vi "Measure_Voltage.vi"(6 "Resolution in Digits":T1(ring), 8 "error in (no error)":errorcluster, 9 "Range":dbl=1.2, 10 "Level":dbl=1.2, 11 "NI-DMM in":refnum<class "niDMM.lvclass">) -> (0 "error out":errorcluster, 1 "Out of Range":bool, 2 "DC_Voltage":dbl, 3 "NI-DMM out":refnum<class "niDMM.lvclass">)   [LabVIEW 2021, in "niDMM.lvclass"]
uses:
  niDMM.lvclass
  niDMM.lvclass/niDMM.ctl
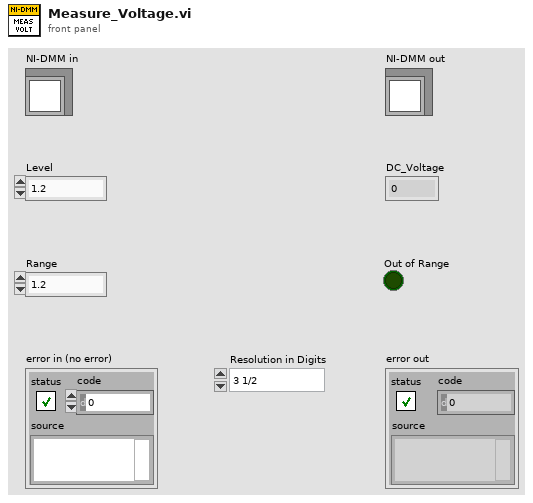
[diagram p1: front panel]
types:
  T1 = enum32{"3 1/2", "4 1/2", "5 1/2", "6 1/2", "7 1/2"}
  T2 = enum32{"DC Volts", "AC Volts", "DC Current", "AC Current", "2-wire Resistance", "4-wire Resistance", "Diode", "Frequency", "Period", "AC Volts DC Coupled", "Capacitance", "Inductance", "Temperature"}
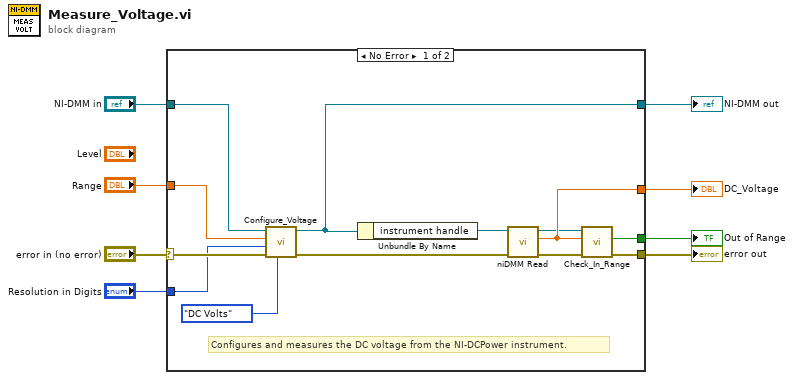
[diagram p0: block diagram]
diagram:
  n1 = case shown="No Error" "error in (no error)" {
    selector: "error in (no error)" -> [w21 w22]
    tunnel: "NI-DMM in" -> [w20 w23]
    tunnel: [w19 w22] -> w6
    tunnel: [w18 _] -> w5
    tunnel: [w15 w23] -> w4
    tunnel: [w16 _] -> w3
    tunnel: "Range" -> [w11 _]
    tunnel: "Resolution in Digits" -> [w10 _]
    frame No Error {
      # "Configures and measures the DC voltage from the NI-DCPower instrument."
      n2 = call-dynamic "Configure_Voltage.vi"("Measurement Type"=T2."DC Volts", "error in (no error)"=w21, "Resolution in Digits"=w10, "Range"=w11, "NI-DMM in"=w20) -> ("error out"=w17:errorcluster, "NI-DMM out"=w15:refnum<class "niDMM.lvclass">)  [unwired: 5 in]
      n3 = Unbundle By Name(w15) -> ("instrument handle"=w14:refnum<k15>)
      n4 = call <instrlib>:"niDMM Read.vi"("error in (no error)"=w17, "instrument handle"=w14) -> ("error out"=w12:errorcluster, "Measurement"=w18:dbl, "instrument handle out"=w13:refnum<k15>)  [unwired: 7 in]
      n5 = call "Check_In_Range.vi"("error in (no error)"=w12, "MeasurementVoltage"=w18, "instrument handle"=w13) -> ("error out"=w19:errorcluster, "Out of Range"=w16:bool)  [unwired: 7 in]
    }
    frame Error {
    }
  }
  "error out" <- w6
  "NI-DMM out" <- w4
  "DC_Voltage" <- w5
  "Out of Range" <- w3
